vi "Set LogEngine Settings.vi"(8 "error in (no error)":errorcluster, 10 "LogEngine Settings":T1, 11 "Config in":refnum<class "Config.lvclass">) -> (0 "error out":errorcluster, 3 "Config out":refnum<class "Config.lvclass">)   [LabVIEW 2019, in "Config.lvclass"]
doc: "Developed by Kevin Thompson\nkevin@thompsonengineering.net\n\nCopyright 2018-2020\nThompson Engineering, LLC"
uses:
  Config.lvclass
  Log_Engine/DataTypes/Settings--cluster.ctl
  Log_Engine/Log_Engine.lvclass
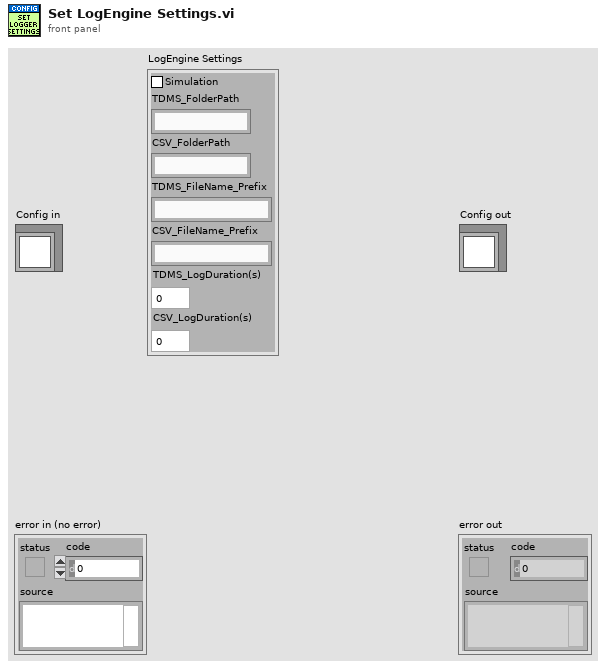
[diagram p1: front panel]
types:
  T1 = typedef "Log_Engine.lvclass/Settings--cluster.ctl" = cluster{"Simulation":bool, "TDMS_FolderPath":string, "CSV_FolderPath":string, "TDMS_FileName_Prefix":string, "CSV_FileName_Prefix":string, "TDMS_LogDuration(s)":dbl, "CSV_LogDuration(s)":dbl}
  T2 = typedef "Config.lvclass/Config Settings.ctl" = cluster{"Application Settings":T3, "Main Settings":T4, "DAQ Settings":T7, "LogEngine Settings":T1}
  T3 = typedef "Application.lvclass/Settings--cluster.ctl" = cluster{"Simulation":bool}
  T4 = typedef "Main.lvclass/Settings--cluster.ctl" = cluster{"Simulation":bool, "Signal scaling":T5, "ESR scaling":T6, "num readings to average":i32, "ESR alarm threshhold (%)":dbl, "UseDummyVrms":bool, "Dummy Vrms":dbl, "Inverter Database File":path, "default Inverter (name)":string}
  T5 = typedef "Main.lvclass/Gain control.ctl" = cluster{"ch0 gain ":dbl, "ch1 gain":dbl, "ch2 gain ":dbl, "ch3 gain ":dbl, "ch0 offest":dbl, "ch1 offset":dbl, "ch2 offset":dbl, "ch3 offset":dbl}
  T6 = typedef "Main.lvclass/ESR scaling--cluster.ctl" = cluster{"Gain":dbl, "Offset":dbl}
  T7 = typedef "DAQ_Engine.lvclass/Settings--cluster.ctl" = cluster{"Simulation":bool, "Initial ErrReporting setting":i32, "Initial Measurement settings":T8, "BoardNum":T10, "Acquisition mode":T11, "DemoMode":bool}
  T8 = typedef "Measurement Config--cluster.ctl" = cluster{"Data Rate 9775":T9, "Data Rate 9215":u32, "Samples RMS 9215":u32, "Samples RMS 9775":u32}
  T9 = typedef "nicrio_cRIO-9775_ContinuousDataRates4ChansRing.ctl" = u16
  T10 = typedef "DAQ_Engine.lvclass/BoardNum--cluster.ctl" = cluster{"P1Sgl":u32, "P2":u32, "P3":u32}
  T11 = typedef "Acquisition Mode--cluster.ctl" = enum16{"3phase", "Single"}
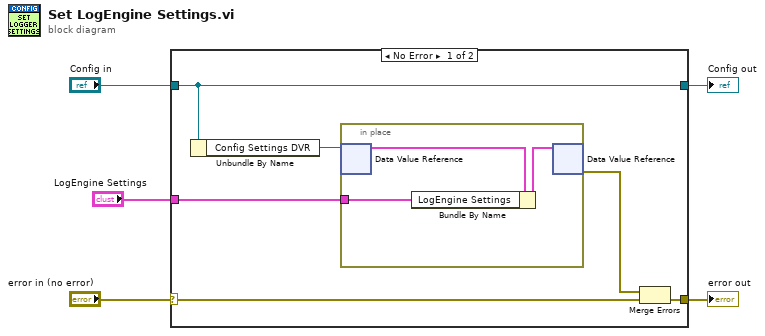
[diagram p0: block diagram]
diagram:
  n1 = case shown="No Error" "error in (no error)" {
    selector: "error in (no error)" -> [w7 w15]
    tunnel: [w6 w15] -> w1
    tunnel: [w9 w16] -> w4
    tunnel: "Config in" -> [w9 w16]
    tunnel: "LogEngine Settings" -> [w8 _]
    frame No Error {
      n2 = Unbundle By Name(w9) -> ("Config Settings DVR"=w11:refnum<data-value>)
      n3 = in-place {
        in-place-border: w8 -> [w12]
        n4 = in-place-dvr #1(w11) -> (w14:T2)  [unwired: 1 out]
        n5 = Bundle By Name(cluster=w14, "LogEngine Settings"=w12) -> (w13:T2)
        n6 = in-place-dvr #1(w13) -> (w10:errorcluster)  [unwired: 1 out]
      }
      n7 = Merge Errors(w10, w7) -> (w6:errorcluster)
    }
    frame Error {
    }
  }
  "error out" <- w1
  "Config out" <- w4
